vi "http add header to set.vi"(6 "continuation?":bool, 7 "override on duplicate?":bool, 9 "header field data":string, 10 "header field name":string, 11 "headers in":T1) -> (3 "headers out":T1)   [LabVIEW 2016, in "http headers.lvlib"]
uses:
  http headers.lvlib
  http header data.ctl
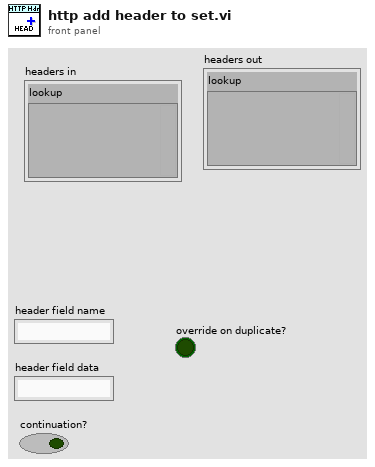
[diagram p1: front panel]
types:
  T1 = typedef "http headers.lvlib/http header data.ctl" = cluster{"lookup":variant}
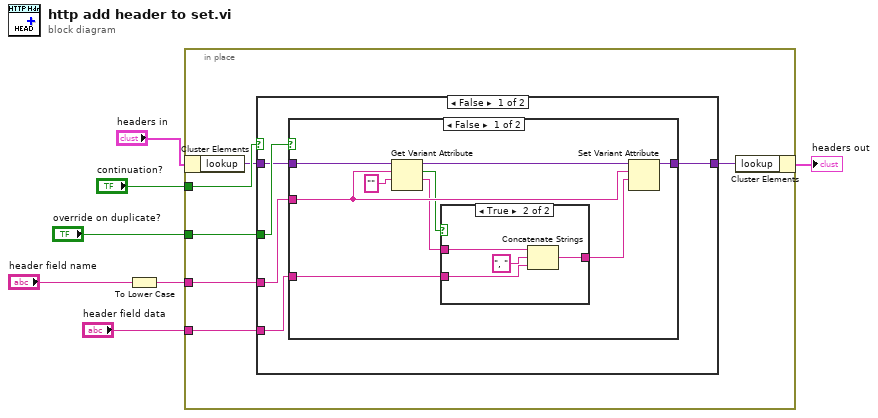
[diagram p0: block diagram]
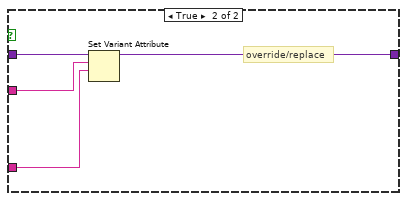
[diagram p3: hidden frame]
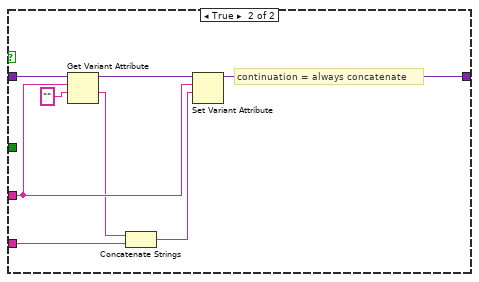
[diagram p4: hidden frame]
diagram:
  n1 = To Lower Case(string="header field name") -> (all lower case string=w1:string)
  n2 = in-place {
    in-place-border: w1 -> [w12]
    in-place-border: "header field data" -> [w13]
    in-place-border: "continuation?" -> [w10]
    in-place-border: "override on duplicate?" -> [w11]
    n3 = in-place-cluster #1("headers in") -> ("lookup"=w9:variant)
    n4 = case shown="False" w10 {
      tunnel: w13 -> [w14 w38]
      tunnel: w12 -> [w15 w43]
      tunnel: w11 -> [w18 _]
      tunnel: w9 -> [w17 w44]
      tunnel: [w16 w41] -> w8
      frame False {
        n5 = case shown="False" w18 {
          tunnel: w17 -> [w25 w36]
          tunnel: [w23 w35] -> w16
          tunnel: w15 -> [w24 w34]
          tunnel: w14 -> [w21 w33]
          frame False {
            n6 = Get Variant Attribute(Variant=w25, name=w24, default value (empty Variant)="") -> (duplicate Variant=w27:variant, found=w20:bool, value=w19:string)  [unwired: 1 in, 1 out]
            n7 = case shown="True" w20 {
              tunnel: [w28 w31] -> w22
              tunnel: w21 -> [w28 w30]
              tunnel: w19 -> [_ w29]
              frame False {
                # "no prior"
              }
              frame True {
                n8 = Concatenate Strings(w29, ", " ("string"), w30) -> (w31:string)
              }
            }
            n9 = Set Variant Attribute(Variant=w27, name=w24, value=w22) -> (Variant out=w23:variant)  [unwired: 1 in, 2 out]
          }
          frame True {
            # "override/replace"
            n10 = Set Variant Attribute(Variant=w36, name=w34, value=w33) -> (Variant out=w35:variant)  [unwired: 1 in, 2 out]
          }
        }
      }
      frame True {
        # "continuation = always concatenate"
        n11 = Get Variant Attribute(Variant=w44, name=w43, default value (empty Variant)="") -> (duplicate Variant=w42:variant, value=w39:string)  [unwired: 1 in, 2 out]
        n12 = Concatenate Strings(w39, w38) -> (w37:string)
        n13 = Set Variant Attribute(Variant=w42, name=w43, value=w37) -> (Variant out=w41:variant)  [unwired: 1 in, 2 out]
      }
    }
    n14 = in-place-cluster #1("lookup"=w8) -> (→"headers out":T1)
  }
